vi "field_to_current_convert.vi"(1 "Field, Oe":dbl) -> (0 "Current, A":dbl)   [LabVIEW 2017]
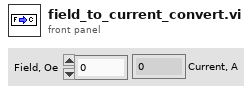
[diagram p1: front panel]
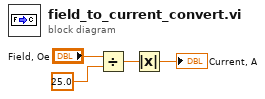
[diagram p0: block diagram]
diagram:
  n1 = Divide(x="Field, Oe", y=25.0) -> (x/y=w2:dbl)
  n2 = Absolute Value(x=w2) -> (abs(x)=→"Current, A":dbl)
